vi "Read data.vi"(0 "VISA resource name":refnum<visa-resource-name>, 5 "Number of samples":i32=-1, 7 "error in (no error)":errorcluster, 8 "Sampling interval, s":dbl=0.000408 format="%_8g") -> (12 "output waveform MA":waveform(dbl), 16 "output array MA":dbl[](array[numeric]) format="%#_10e", 20 "VISA resource name out":refnum<visa-resource-name>, 27 "error out Master":errorcluster)   [LabVIEW 2020, in "3458A Virtual Digitizer.lvlib" / "3458A Digitizing Low Levels.lvlib"]
doc: "This VI reads the data from the instrument´s memory, it then outputs the waveform for the input of the data processing module."
uses:
  3458A Digitizing Low Levels.lvlib
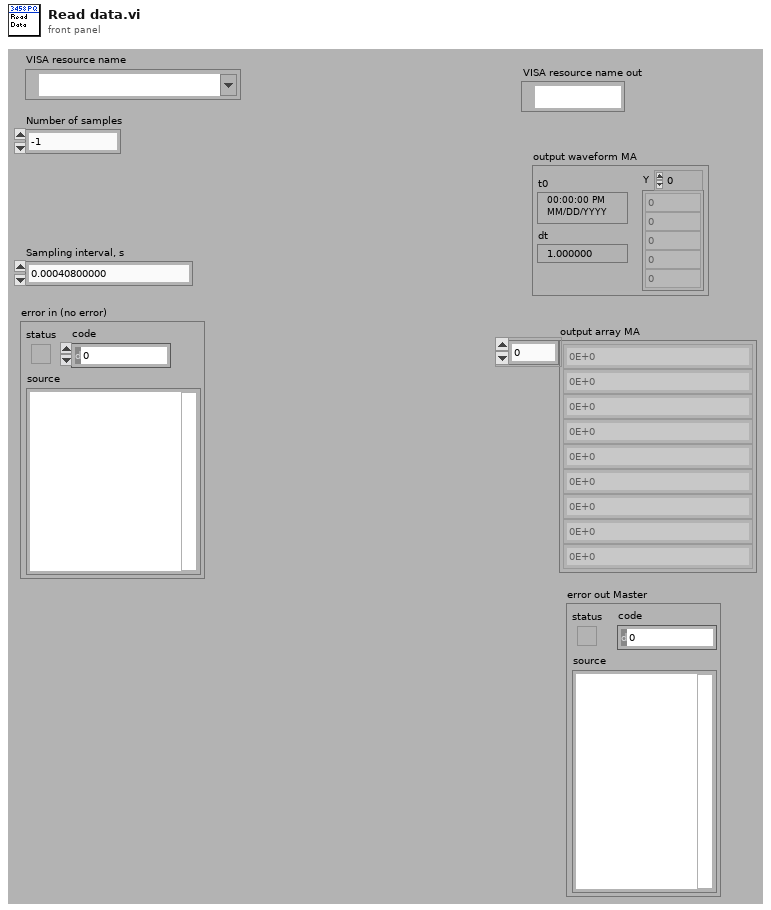
[diagram p1: front panel]
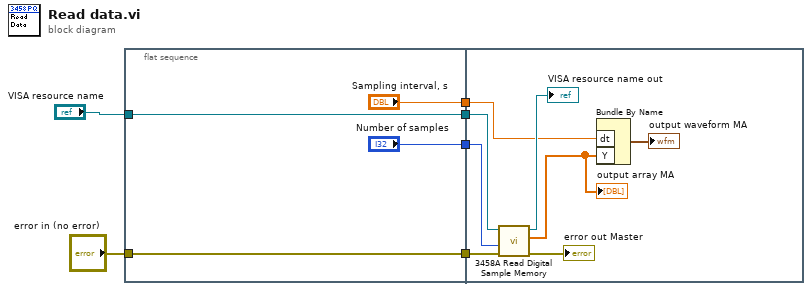
[diagram p0: block diagram]
diagram:
  n1 = flat-sequence {
    tunnel: [w10] -> w6
    tunnel: "error in (no error)" -> [w10]
    tunnel: [w9] -> w4
    tunnel: "VISA resource name" -> [w9]
    tunnel: ["Sampling interval, s"] -> w2
    tunnel: ["Number of samples"] -> w1
    tunnel: w6 -> [w15]
    tunnel: w4 -> [w16]
    tunnel: w2 -> [w12]
    tunnel: w1 -> [w14]
    frame #0 {
    }
    frame #1 {
      n2 = call "3458A Read Digital Sample Memory.vi"("error in (no error)"=w15, "max read [smpl]"=w14, "VISA session"=w16) -> ("error out"=→"error out Master":errorcluster, "waveform data [V]"=w11:dbl[], "dup VISA session"=→"VISA resource name out":refnum<visa-resource-name>)  [unwired: 2 in, 4 out]
      "output array MA" <- w11
      n3 = Bundle By Name("dt"=w12, "Y"=w11) -> (→"output waveform MA":waveform(dbl))  [unwired: 1 in]
    }
  }
